vi "Get Array Element Offsets.vi"(8 "error in (no error)":errorcluster, 9 "Max Index":i32=2147483647, 10 "Offset":i32, 11 "JSON":string="[1,2,3]") -> (0 "error out":errorcluster, 1 "Elements":T1[](array[typedef]), 2 "Offset past Array":i32, 4 "Comma Needed for Insert":bool)   [LabVIEW 2019, in "JSONtext.lvlib"]
uses:
  JSONtext.lvlib
  Parsing/Found Items.ctl
  Parsing/Parsing State.ctl
  Parsing/Advance past Line Ending.vi
  Parsing/Advance past String.vi
  Parsing/Advance past Number.vi
  Parsing/Advance past Array.vi
  Parsing/Advance past Object.vi
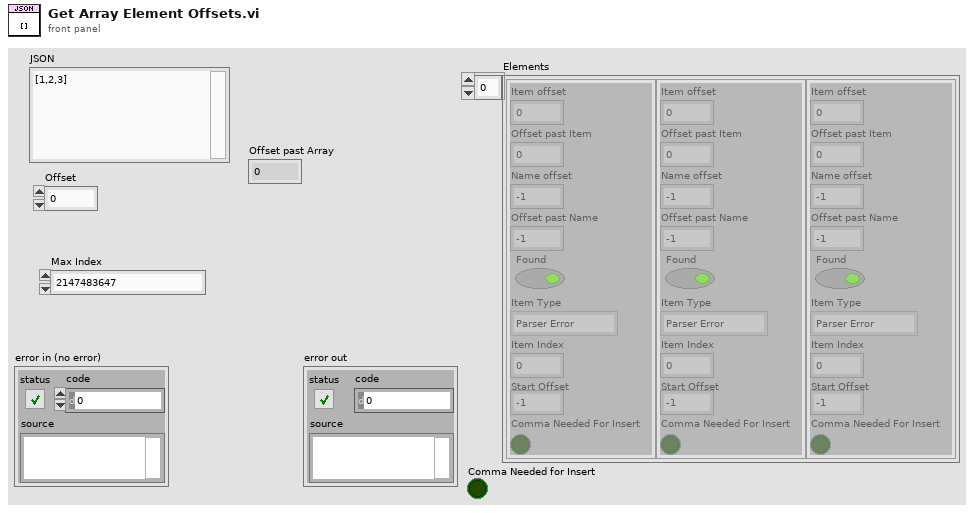
[diagram p1: front panel]
types:
  T1 = typedef "JSONtext.lvlib/Found Items.ctl" = cluster{"Item offset":i32, "Offset past Item":i32, "Name offset":i32, "Offset past Name":i32, "Found":bool, "Item Type":T2, "Item Index":i32, "Start Offset":i32, "Comma Needed For Insert":bool}
  T2 = typedef "JSONtext.lvlib/Parsing State.ctl" = enum16{"Parser Error", "Object", "Array", "String", "Number/Other", "Leading Whitespace", "Object end", "Array end", "Value end"}
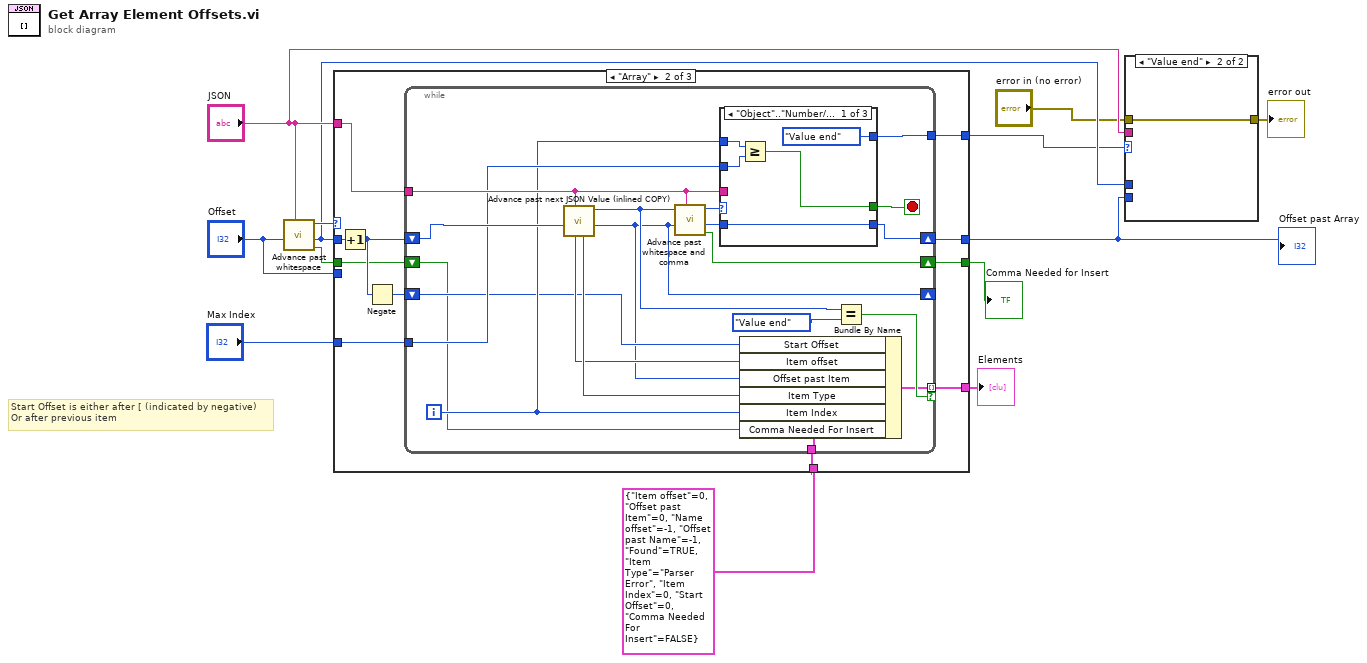
[diagram p0: block diagram]
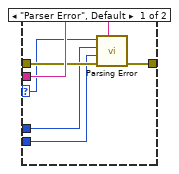
[diagram p2: hidden frame]
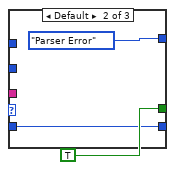
[diagram p4: hidden frame]
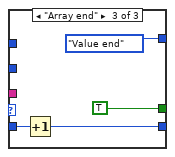
[diagram p5: hidden frame]
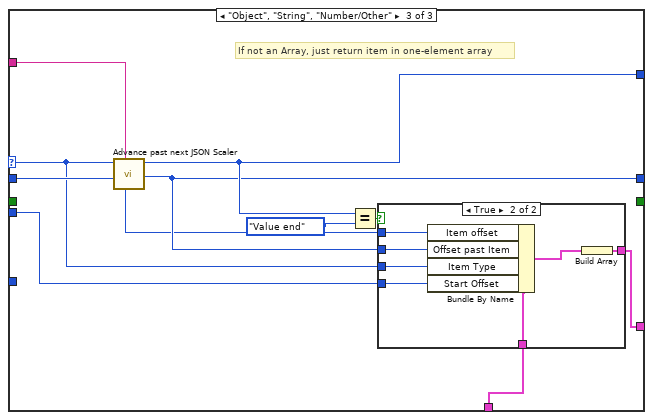
[diagram p6: hidden frame]
diagram:
  # "Start Offset is either after [ (indicated by negative)\nOr after previous item"
  n1 = call "Advance past whitespace.vi"("JSON"="JSON", "Offset"="Offset") -> ("Comma Not Found"=w2:bool, "Offset of first non-whitespace"=w11:i32, "Parser State"=w13:T2)  [unwired: 7 in]
  n2 = case shown="\"Array\"" w13 {
    selector: w13 -> [w15 _ w62]
    tunnel: [w15 w26 w66] -> w7
    tunnel: [w14 w25 w61] -> w10
    tunnel: [_ w24 w64] -> w6
    tunnel: "JSON" -> [_ w23 w67]
    tunnel: w11 -> [w14 w22 w69]
    tunnel: "Max Index" -> [_ w21 _]
    tunnel: T1 {"Item offset"=0, "Offset past Item"=0, "Name offset"=-1, "Offset past Name"=-1, "Found"=TRUE, "Item Type"=enum."Parser Error", "Item Index"=0, "Start Offset"=0, "Comma Needed For Insert"=FALSE} -> [_ w20 w63]
    tunnel: "Offset" -> [_ _ w59]
    tunnel: w2 -> [_ w17 _]
    tunnel: [_ w16 _] -> w1
    frame "Parser Error", Default {
    }
    frame "Array" {
      n3 = Increment(x=w22) -> (x+1=w19:i32)
      n4 = Negate(x=w19) -> (-x=w18:i32)
      n5 = while {
        tunnel: w23 -> [w40]
        shift-right: [w43] -> w25
        shift-left: w19 -> [w44]
        tunnel: [w41] -> w26
        tunnel: [w31] -> w24 mode=indexing if=w37
        tunnel: w21 -> [w36]
        tunnel: w20 -> [w35]
        shift-right: [w29] -> _
        shift-left: w18 -> [w30]
        shift-right: [w28] -> w16
        shift-left: w17 -> [w27]
        i -> [w34]
        stop <- w42 stop-if-true
        n6 = call "Advance past next JSON Value (inlined COPY).vi"("JSON"=w40, "Offset"=w44) -> ("Offset"=w29:i32, "State"=w38:T2, "Type"=w33:T2, "Value start"=w32:i32)  [unwired: 5 in, 1 out]
        n7 = call "Advance past whitespace and comma.vi"("JSON"=w40, "Offset"=w29, "State in"=w38) -> ("Comma Not Found"=w28:bool, "Offset past match"=w46:i32, "State"=w45:T2)  [unwired: 6 in]
        n8 = case shown="\"Object\"..\"Number/Other\"" w45 {
          tunnel: [w48 TRUE TRUE] -> w42
          tunnel: [Parsing_State."Value end" Parsing_State."Parser Error" Parsing_State."Value end"] -> w41
          tunnel: w46 -> [w51 w52 w56]
          tunnel: [w51 w52 w55] -> w43
          tunnel: w40 -> [_ _ _]
          tunnel: w34 -> [w49 _ _]
          tunnel: w36 -> [w50 _ _]
          frame "Object".."Number/Other" {
            n9 = Greater Or Equal?(x=w49, y=w50) -> (x >= y?=w48:bool)
          }
          frame Default {
          }
          frame "Array end" {
            n10 = Increment(x=w56) -> (x+1=w55:i32)
          }
        }
        n11 = Bundle By Name(cluster=w35, "Start Offset"=w30, "Item offset"=w32, "Offset past Item"=w29, "Item Type"=w33, "Item Index"=w34, "Comma Needed For Insert"=w27) -> (w31:T1)
        n12 = Equal?(x=w38, y=Parsing_State."Value end") -> (x = y?=w37:bool)
      }
    }
    frame "Object", "String", "Number/Other" {
      # "If not an Array, just return item in one-element array"
      n13 = call "Advance past next JSON Scaler.vi"("JSON"=w67, "Offset"=w69, "Parser State in"=w62) -> ("Offset Past"=w61:i32, "Parser State"=w66:T2, "Value start"=w60:i32)  [unwired: 6 in]
      n14 = Equal?(x=w66, y=Parsing_State."Value end") -> (x = y?=w65:bool)
      n15 = case shown="True" w65 {
        tunnel: [_ w76] -> w64
        tunnel: w63 -> [_ w75]
        tunnel: w62 -> [_ w74]
        tunnel: w61 -> [_ w73]
        tunnel: w60 -> [_ w72]
        tunnel: w59 -> [_ w70]
        frame False {
        }
        frame True {
          n16 = Bundle By Name(cluster=w75, "Item offset"=w72, "Offset past Item"=w73, "Item Type"=w74, "Start Offset"=w70) -> (w71:T1)
          n17 = Build Array(w71) -> (w76:T1[])
        }
      }
    }
  }
  "Offset past Array" <- w10
  "Elements" <- w6
  "Comma Needed for Insert" <- w1
  n18 = case shown="\"Value end\"" w7 {
    selector: w7 -> [w77 _]
    tunnel: "JSON" -> [w82 _]
    tunnel: "error in (no error)" -> [w81 w83]
    tunnel: [w80 w83] -> w9
    tunnel: w11 -> [w79 _]
    tunnel: w10 -> [w78 _]
    frame "Parser Error", Default {
      n19 = call "Parsing Error.vi"("JSON"=w82, "error in (no error)"=w81, "Offset past match"=w78, "Value start"=w79, "State"=w77) -> ("error out"=w80:errorcluster)  [unwired: 6 in]
    }
    frame "Value end" {
    }
  }
  "error out" <- w9
